vi "setEMGain.vi"(6 "Delay between send and receive [ms]":i32=100, 8 "error in (no error)":errorcluster, 10 "gain":i32, 11 "CCD in":refnum<class "CCD.lvclass">) -> (0 "error out":errorcluster, 1 "ID":i32, 2 "results-JSON string":string, 3 "CCD out":refnum<class "CCD.lvclass">)   [LabVIEW 2020, in "horiba.lvlib" / "CCD.lvclass"]
doc: "Sets the CCD gain token. A list of supported gain tokens can be found in the CCD configuration. See ccd_getConfig command.\nFor example:\n\n\"gains\": [\n {\n \"info\": \"Best Dynamic Range\",\n \"token\": 1\n },\n {\n \"info\": \"High Sensitivity\",\n \"token\": 2\n },\n {\n \"info\": \"High Light\",\n \"token\": 0\n }\n]"
uses:
  CCD.lvclass
  <vilib>/JDP Science/JSONtext/LVClass Serializer/JSONtext LVClass Serializer.lvclass
  20f7d3bd-08ac-4524-9bed-df36c1da25a0.vi
  GenericDevice/GenericDevice.lvclass
  5b02aa1a-f403-4d30-91c8-1c594f70e61d.vi
panel:
  # "Connector Pane"
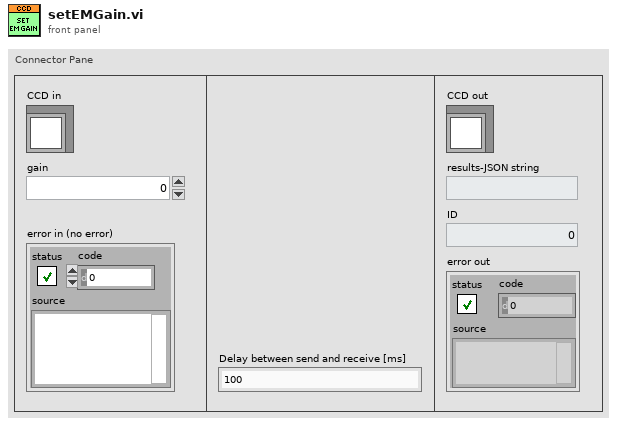
[diagram p1: front panel]
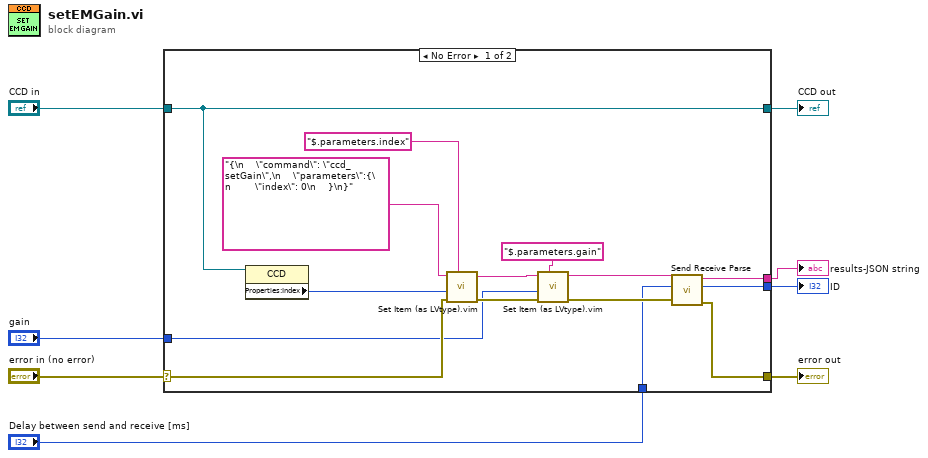
[diagram p0: block diagram]
diagram:
  n1 = case shown="No Error" "error in (no error)" {
    selector: "error in (no error)" -> [w20 w25]
    tunnel: [w16 w25] -> w7
    tunnel: [w11 w24] -> w5
    tunnel: "CCD in" -> [w11 w24]
    tunnel: [w14 _] -> w4
    tunnel: [w15 _] -> w3
    tunnel: "Delay between send and receive [ms]" -> [w10 _]
    tunnel: "gain" -> [w9 _]
    frame No Error {
      n2 = property class="CCD"(reference=w11) -> ("Properties:Index"=w21:i32)  [unwired: 1 in, 2 out]
      n3 = call "Set Item (as LVtype).vim"("$Path or Item Name"="$.parameters.index", "error in (no error)"=w20, "Anything"=w21, "JSON"="{\n    \"command\": \"ccd_setGain\",\n    \"parameters\":{\n        \"index\": 0\n    }\n}") -> ("error out"=w12:errorcluster, "<JSON>"=w19:string)  [unwired: 4 in, 1 out]
      n4 = call "Set Item (as LVtype).vim"("$Path or Item Name"="$.parameters.gain", "error in (no error)"=w12, "Anything"=w9, "JSON"=w19) -> ("error out"=w18:errorcluster, "<JSON>"=w13:string)  [unwired: 4 in, 1 out]
      n5 = call "Send Receive Parse.vi"("error in"=w18, "Delay between send and receive [ms]"=w10, "<JSON>"=w13) -> ("error out"=w16:errorcluster, "ID"=w15:i32, "results-JSON string"=w14:string)  [unwired: 6 in]
    }
    frame Error {
    }
  }
  "error out" <- w7
  "CCD out" <- w5
  "results-JSON string" <- w4
  "ID" <- w3
